vi "Inst.AH2500.getAll.vi"(8 "error in (no error)":errorcluster, 11 "Inst.AH2500 in":refnum<class "Inst.AH2500.lvclass">) -> (0 "error out":errorcluster, 2 "output cluster":T1, 3 "Inst.AH2500 out":refnum<class "Inst.AH2500.lvclass">)   [LabVIEW 2019, in "Inst.AH2500.lvclass"]
uses:
  Inst.AH2500.lvclass
  Typedefs/Inst.AH2500.getAll--Cluster.ctl
  Inst.AH2500.lvclass/Inst.AH2500.ctl
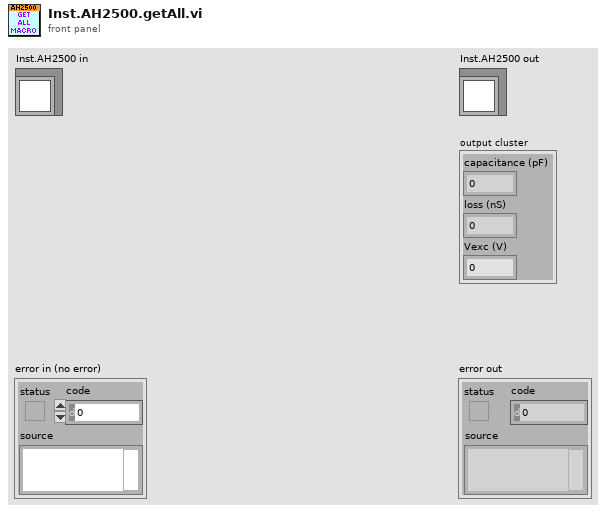
[diagram p1: front panel]
types:
  T1 = typedef "Inst.AH2500.lvclass/Inst.AH2500.getAll--Cluster.ctl" = cluster{"capacitance (pF)":dbl, "loss (nS)":dbl, "Vexc (V)":dbl}
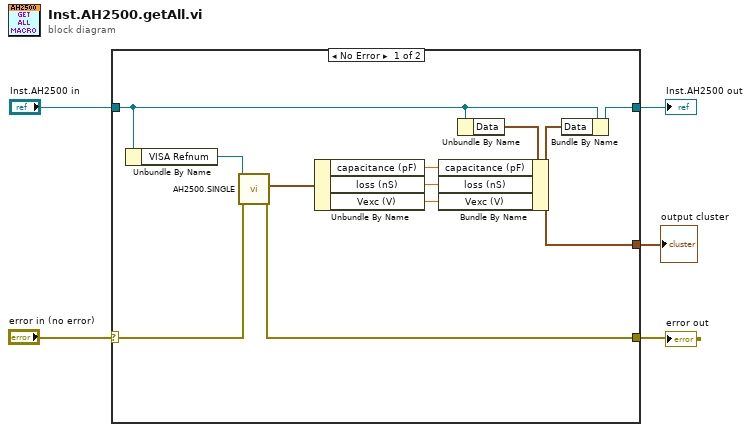
[diagram p0: block diagram]
diagram:
  n1 = case shown="No Error" "error in (no error)" {
    selector: "error in (no error)" -> [w7 w18]
    tunnel: [w6 w18] -> w3
    tunnel: [w15 w17] -> w2
    tunnel: "Inst.AH2500 in" -> [w14 w17]
    tunnel: [w13 _] -> w1
    frame No Error {
      n2 = Unbundle By Name(w14) -> ("VISA Refnum"=w12:refnum<visa-resource-name>)
      n3 = call "AH2500.SINGLE.vi"("error in (no error)"=w7, "VISA resource name"=w12) -> ("error out"=w6:errorcluster, "Measurement"=w11:T1)  [unwired: 7 in, 1 out]
      n4 = Unbundle By Name(w11) -> ("capacitance (pF)"=w10:dbl, "loss (nS)"=w9:dbl, "Vexc (V)"=w8:dbl)
      n5 = Unbundle By Name(w14) -> ("Data"=w16:T1)
      n6 = Bundle By Name(cluster=w16, "capacitance (pF)"=w10, "loss (nS)"=w9, "Vexc (V)"=w8) -> (w13:T1)
      n7 = Bundle By Name(cluster=w14, "Data"=w13) -> (w15:refnum<class "Inst.AH2500.lvclass">)
    }
    frame Error {
    }
  }
  "error out" <- w3
  "Inst.AH2500 out" <- w2
  "output cluster" <- w1
